vi "Set Clock Source.vi"(0 "Arduino Resource":T1={"VISA resource"="", "Board Type"=enum."Uno", "Connection Type"=enum."USB / Serial", "Bytes Per Packet (15)"=15}, 5 "Device Address":T3=104 items=["0x68"=104, "0x69"=105], 9 "Clock Source":u8, 11 "error in (no error)":errorcluster) -> (4 "Arduino Resource":T1={"VISA resource"="", "Board Type"=enum."Uno", "Connection Type"=enum."USB / Serial", "Bytes Per Packet (15)"=15}, 15 "error out":errorcluster)   [LabVIEW 2016, in "LIFA MPU-60X0.lvlib"]
doc: "Sets the clock source.\n\n0 - Internal 8MHz oscillator\n1 - PLL with X axis gyroscope reference\n2 - PLL with Y axis gyroscope reference\n3 - PLL with Z axis gyroscope reference\n4 - PLL with external 32.768kHz reference\n5 - PLL with external 19.2MHz reference\n6 - Reserved\n7 - Stops the clock and keeps the timing generator in reset"
uses:
  LIFA MPU-60X0.lvlib
  RegisterAddresses.ctl
  DeviceAddresses.ctl
  <vilib>/LabVIEW Interface for Arduino/Type Defs/Board Type.ctl
  <vilib>/LabVIEW Interface for Arduino/Type Defs/Arduino Resource.ctl
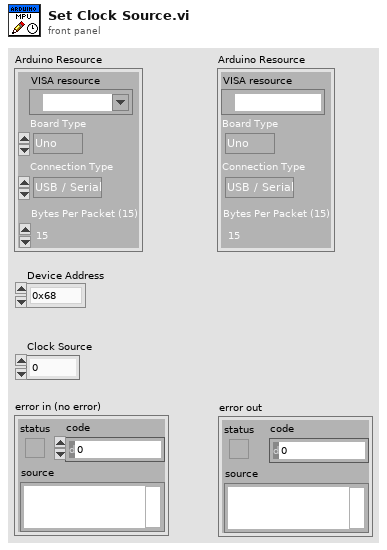
[diagram p1: front panel]
types:
  T1 = typedef "LabVIEW Interface for Arduino.lvlib/Arduino Resource.ctl" = cluster{"VISA resource":refnum<visa-resource-name>, "Board Type":T2, "Connection Type":enum8{"USB / Serial"}, "Bytes Per Packet (15)":u8}
  T2 = typedef "LabVIEW Interface for Arduino.lvlib/Board Type.ctl" = enum16{"Uno", "Dimuelanove w/Atmega 328", "Mega 2560"}
  T3 = typedef "LIFA MPU-60X0.lvlib/DeviceAddresses.ctl" = u8
  T4 = typedef "LIFA MPU-60X0.lvlib/RegisterAddresses.ctl" = u16
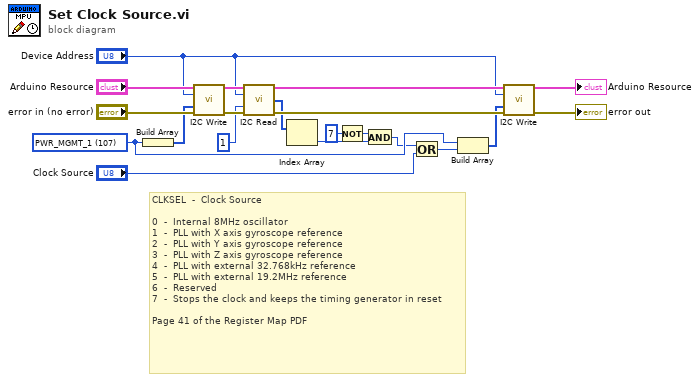
[diagram p0: block diagram]
diagram:
  w10 = T4 107 items=["SELF_TEST_X"=13, "SELF_TEST_Y"=14, "SELF_TEST_Z"=15, "SELF_TEST_A"=16, "SMPLRT_DIV"=25, "CONFIG"=26, "GYRO_CONFIG"=27, "ACCEL_CONFIG"=28, "MOT_THR"=31, "FIFO_EN"=35, "I2C_MST_CTRL"=36, "I2C_SLV0_ADDR"=37, "I2C_SLV0_REG"=38, "I2C_SLV0_CTRL"=39, "I2C_SLV1_ADDR"=40, "I2C_SLV1_REG"=41, "I2C_SLV1_CTRL"=42, "I2C_SLV2_ADDR"=43, "I2C_SLV2_REG"=44, "I2C_SLV2_CTRL"=45, "I2C_SLV3_ADDR"=46, "I2C_SLV3_REG"=47, "I2C_SLV3_CTRL"=48, "I2C_SLV4_ADDR"=49, "I2C_SLV4_REG"=50, "I2C_SLV4_DO"=51, "I2C_SLV4_CTRL"=52, "I2C_SLV4_DI"=53, "I2C_MST_STATUS"=54, "INT_PIN_CFG"=55, "INT_ENABLE"=56, "INT_STATUS"=58, "ACCEL_XOUT_H"=59, "ACCEL_XOUT_L"=60, "ACCEL_YOUT_H"=61, "ACCEL_YOUT_L"=62, "ACCEL_ZOUT_H"=63, "ACCEL_ZOUT_L"=64, "TEMP_OUT_H"=65, "TEMP_OUT_L"=66, "GYRO_XOUT_H"=67, "GYRO_XOUT_L"=68, "GYRO_YOUT_H"=69, "GYRO_YOUT_L"=70, "GYRO_ZOUT_H"=71, "GYRO_ZOUT_L"=72, "EXT_SENS_DATA_00"=73, "EXT_SENS_DATA_01"=74, "EXT_SENS_DATA_02"=75, "EXT_SENS_DATA_03"=76, "EXT_SENS_DATA_04"=77, "EXT_SENS_DATA_05"=78, "EXT_SENS_DATA_06"=79, "EXT_SENS_DATA_07"=80, "EXT_SENS_DATA_08"=81, "EXT_SENS_DATA_09"=82, "EXT_SENS_DATA_10"=83, "EXT_SENS_DATA_11"=84, "EXT_SENS_DATA_12"=85, "EXT_SENS_DATA_13"=86, "EXT_SENS_DATA_14"=87, "EXT_SENS_DATA_15"=88, "EXT_SENS_DATA_16"=89, "EXT_SENS_DATA_17"=90, "EXT_SENS_DATA_18"=91, "EXT_SENS_DATA_19"=92, "EXT_SENS_DATA_20"=93, "EXT_SENS_DATA_21"=94, "EXT_SENS_DATA_22"=95, "EXT_SENS_DATA_23"=96, "I2C_SLV0_DO"=99, "I2C_SLV1_DO"=100, "I2C_SLV2_DO"=101, "I2C_SLV3_DO"=102, "I2C_MST_DELAY_CTRL"=103, "SIGNAL_PATH_RESET"=104, "MOT_DETECT_CTRL"=105, "USER_CTRL"=106, "PWR_MGMT_1"=107, "PWR_MGMT_2"=108, "FIFO_COUNTH"=114, "FIFO_COUNTL"=115, "FIFO_R_W"=116, "WHO_AM_I"=117] ("Register Addresses")
  # "CLKSEL  -  Clock Source\n\n0  -  Internal 8MHz oscillator\n1  -  PLL with X axis gyroscope reference\n2  -  PLL with Y axis gyroscope reference\n3  -  PLL with Z axis gyroscope reference\n4  -  PLL with external 32.768kHz reference\n5  -  PLL with external 19.2MHz reference\n6  -  Reserved\n7  -  Stops the clock and keeps the timing generator in reset\n\nPage 41 of the Register Map PDF"
  n1 = Build Array(w10) -> (w13:T4[])
  n2 = call <vilib>:"I2C Write.vi"("Arduino Resource"="Arduino Resource", "Address (0)"="Device Address", "I2C Data Bytes"=w13, "error in"="error in (no error)") -> ("Arduino Resource"=w20:T1, "error out"=w19:errorcluster)  [unwired: 10 in]
  n3 = call <vilib>:"I2C Read.vi"("Arduino Resource"=w20, "Address (0)"="Device Address", "Bytes To Read"=u8 1, "error in"=w19) -> ("Arduino Resource"=w17:T1, "I2C Data"=w12:u8[], "error out"=w18:errorcluster)  [unwired: 9 in]
  n4 = Index Array(array=w12) -> (element=w5:u8)  [unwired: 1 in]
  n5 = Not(x=u8 7) -> (.not. x?=w4:u8)
  n6 = And(x=w4, y=w5) -> (x .and. y?=w2:u8)
  n7 = Or(x=w2, y="Clock Source") -> (x .or. y?=w11:u8)
  n8 = Build Array(w10, w11) -> (w9:T4[])
  n9 = call <vilib>:"I2C Write.vi"("Arduino Resource"=w17, "Address (0)"="Device Address", "I2C Data Bytes"=w9, "error in"=w18) -> ("Arduino Resource"=→"Arduino Resource":T1, "error out"=→"error out":errorcluster)  [unwired: 10 in]
